vi "Traverse Category Tree.vi"(8 "error in (no error)":errorcluster, 10 "String In":string, 11 "Category in":refnum<class "Category.lvclass">) -> (0 "error out":errorcluster, 2 "String Out":string, 3 "Category out":refnum<class "Category.lvclass">)   [LabVIEW 2013, in "Category.lvclass"]
uses:
  Category.lvclass
  Categories/Categories.lvclass
  xCE/xceNode/xceNode.lvclass
  xCE/xceDataNode/xceDataNode.lvclass
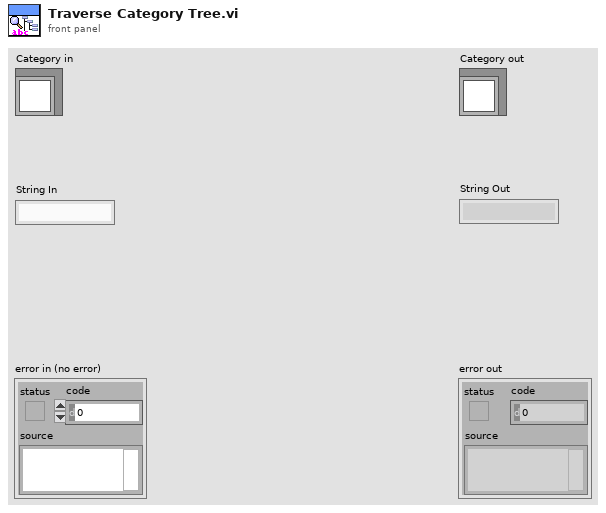
[diagram p1: front panel]
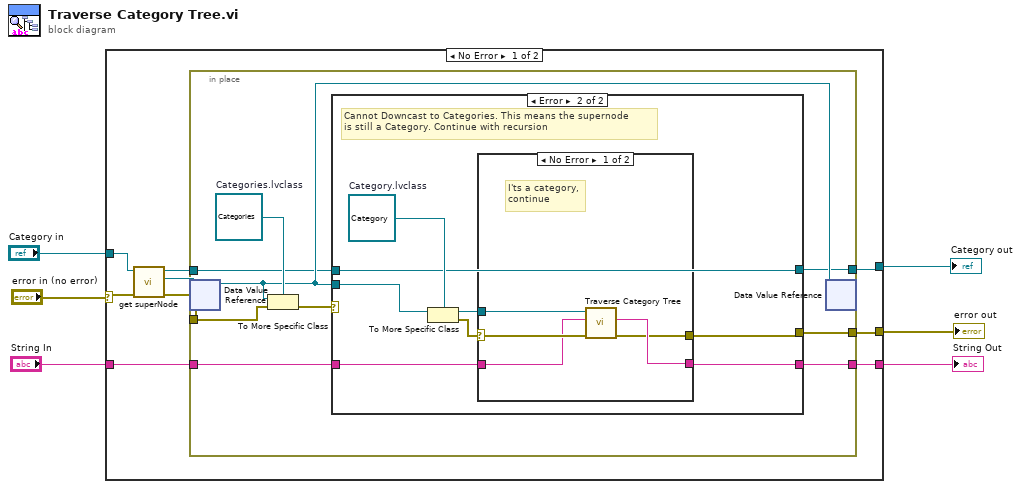
[diagram p0: block diagram]
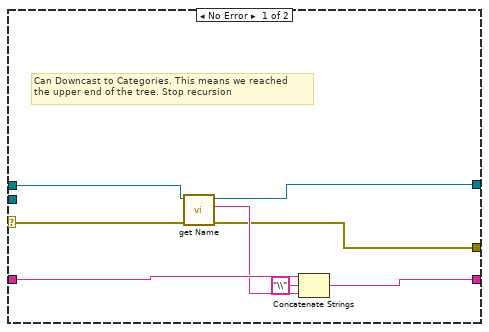
[diagram p2: hidden frame]
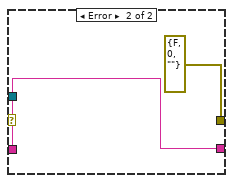
[diagram p3: hidden frame]
diagram:
  n1 = case shown="No Error" "error in (no error)" {
    selector: "error in (no error)" -> [w14 w50]
    tunnel: [w11 w50] -> w2
    tunnel: "Category in" -> [w15 w48]
    tunnel: "String In" -> [w13 w49]
    tunnel: [w12 w49] -> w3
    tunnel: [w7 w48] -> w1
    frame No Error {
      n2 = call "get superNode.vi"("error in (no error)"=w14, "xceNode in"=w15) -> ("error out"=w9:errorcluster, "superNode*"=w10:refnum<data-value>, "xceNode out"=w8:refnum<class "Category.lvclass">)  [unwired: 7 in]
      n3 = in-place {
        in-place-border: w13 -> [w24]
        in-place-border: [w23] -> w12
        in-place-border: [w22] -> w11
        in-place-border: w9 -> [w19]
        in-place-border: w8 -> [w17]
        in-place-border: [w16] -> w7
        w21 = refnum<class "Categories.lvclass"> refnum  # Categories.lvclass
        n4 = in-place-dvr #1(w10) -> (w18:refnum<class "xceTreeObj.lvclass">)  [unwired: 1 out]
        n5 = To More Specific Class(target class=w21, reference=w18, error in=w19) -> (error out=w20:errorcluster)  [unwired: 1 out]
        n6 = case shown="Error" w20 {
          selector: w20 -> [w25 _]
          tunnel: w24 -> [w32 w40]
          tunnel: [w31 w39] -> w23
          tunnel: [w28 w34] -> w22
          tunnel: w18 -> [_ w36]
          tunnel: w17 -> [w27 w33]
          tunnel: [w26 w33] -> w16
          frame No Error {
            # "Can Downcast to Categories. This means we reached\nthe upper end of the tree. Stop recursion"
            n7 = call "get Name.vi"("error in (no error)"=w25, "xceDataNode in"=w27) -> ("error out"=w28:errorcluster, "Name"=w30:string, "xceDataNode out"=w26:refnum<class "Category.lvclass">)  [unwired: 7 in]
            n8 = Concatenate Strings(w32, "\\" ("string"), w30) -> (w31:string)
          }
          frame Error {
            w35 = refnum<class "Category.lvclass"> refnum  # Category.lvclass
            # "Cannot Downcast to Categories. This means the supernode\nis still a Category. Continue with recursion"
            n9 = To More Specific Class(target class=w35, reference=w36) -> (specific class reference=w37:refnum<class "Category.lvclass">, error out=w38:errorcluster)  [unwired: 1 in]
            n10 = case shown="No Error" w38 {
              selector: w38 -> [w45 _]
              tunnel: w40 -> [w44 w47]
              tunnel: [w43 w47] -> w39
              tunnel: [w42 errorcluster {"status"=FALSE, "code"=0, "source"=""} ("error out")] -> w34
              tunnel: w37 -> [w41 _]
              frame No Error {
                # "I'ts a category,\ncontinue"
                n11 = call "Traverse Category Tree.vi"("error in (no error)"=w45, "String In"=w44, "Category in"=w41) -> ("error out"=w42:errorcluster, "String Out"=w43:string)  [unwired: 6 in, 1 out]
              }
              frame Error {
              }
            }
          }
        }
        n12 = in-place-dvr #1(w18) -> ()  [unwired: 2 out]
      }
    }
    frame Error {
    }
  }
  "error out" <- w2
  "Category out" <- w1
  "String Out" <- w3
